vi "HTML_ArrayToTableContent.vi"(7 "<th> (T) / <td> (F)":bool, 10 "Table foot[2D]":string[][](array[string])) -> (2 "resulting string":string)   [LabVIEW 2014]
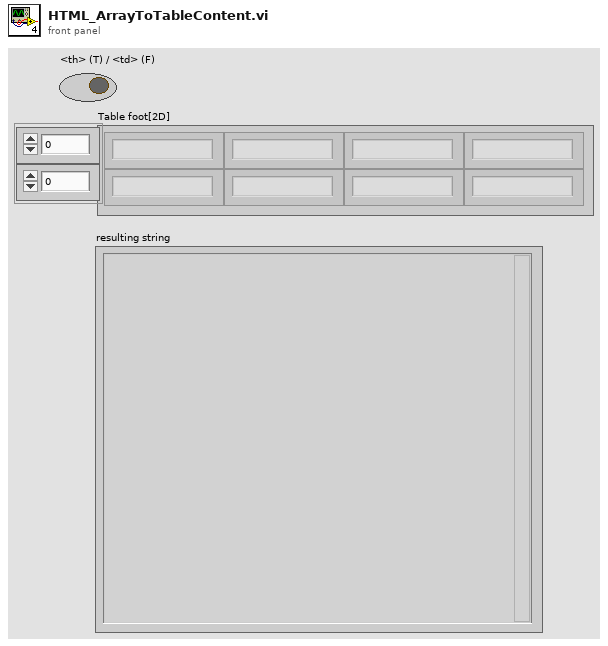
[diagram p1: front panel]
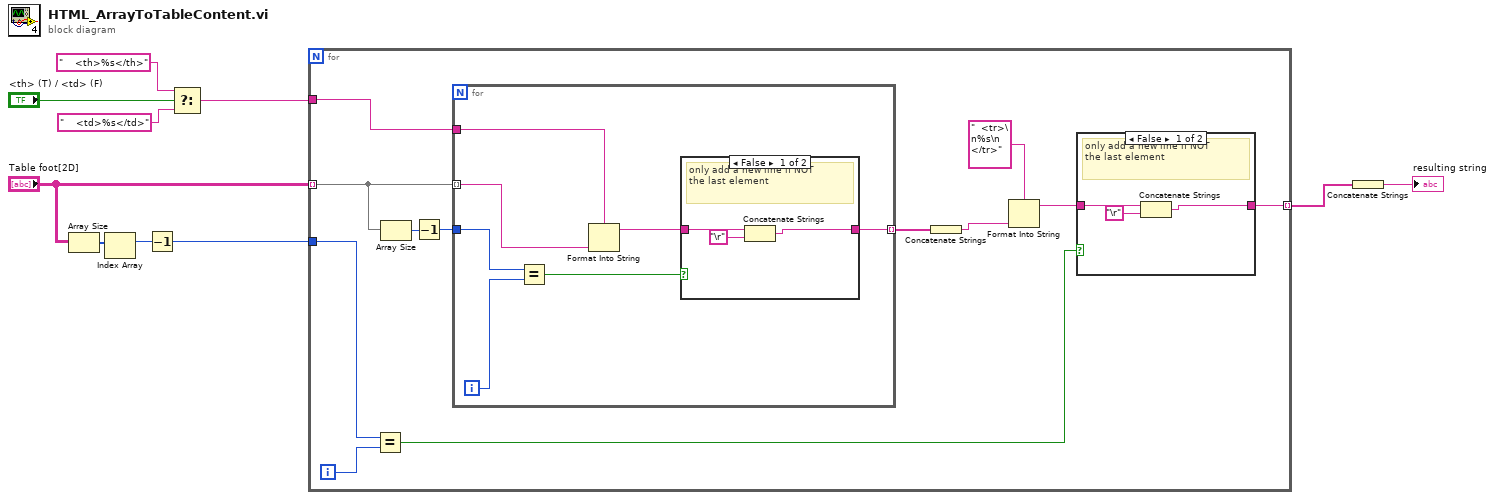
[diagram p0: block diagram]
diagram:
  n1 = Array Size(array="Table foot[2D]") -> (size(s)=w8:i32[])
  n2 = Index Array(array=w8) -> (element=w7:i32)  [unwired: 1 in]
  n3 = Decrement(x=w7) -> (x-1=w5:i32)
  n4 = Select(t="    <th>%s</th>" ("format string"), s="<th> (T) / <td> (F)", f="    <td>%s</td>" ("format string")) -> (s? t:f=w1:string)
  n5 = for {
    tunnel: "Table foot[2D]" -> [w19] mode=indexing
    tunnel: [w13] -> w10 mode=indexing
    tunnel: w5 -> [w16]
    tunnel: w1 -> [w12]
    i -> [w15]
    n6 = Equal?(x=w16, y=w15) -> (x = y?=w11:bool)
    n7 = Array Size(array=w19) -> (size(s)=w18:i32)
    n8 = Decrement(x=w18) -> (x-1=w17:i32)
    n9 = for {
      tunnel: w19 -> [w33] mode=indexing
      tunnel: [w29] -> w21 mode=indexing
      tunnel: w17 -> [w32]
      tunnel: w12 -> [w27]
      i -> [w31]
      n10 = Equal?(x=w32, y=w31) -> (x = y?=w28:bool)
      n11 = Format Into String(format string=w27, w33) -> (resulting string=w30:string)  [unwired: 2 in, 1 out]
      n12 = case shown="False" w28 {
        tunnel: w30 -> [w36 w37]
        tunnel: [w35 w37] -> w29
        frame False {
          # "only add a new line if NOT\nthe last element"
          n13 = Concatenate Strings(w36, "\r") -> (w35:string)
        }
        frame True {
        }
      }
    }
    n14 = Concatenate Strings(w21) -> (w20:string)
    n15 = Format Into String(format string="  <tr>\n%s\n  </tr>", w20) -> (resulting string=w14:string)  [unwired: 2 in, 1 out]
    n16 = case shown="False" w11 {
      tunnel: w14 -> [w25 w26]
      tunnel: [w24 w26] -> w13
      frame False {
        # "only add a new line if NOT\nthe last element"
        n17 = Concatenate Strings(w25, "\r") -> (w24:string)
      }
      frame True {
      }
    }
  }
  n18 = Concatenate Strings(w10) -> (→"resulting string":string)
